vi "DllFxpAtan2Temp.vi"(6 "ready for output":bool, 9 "input valid":bool, 10 "x":fxp<+/-,64,32>, 11 "y":fxp<+/-,64,32>) -> (1 "output valid":bool, 3 "atan2(y, x)":fxp<+,1,1>, 4 "ready for input":bool)   [LabVIEW 2017]
uses:
  <vilib>/rvi/FXPMathLib/FxpAtan2/subVIs/nifxpmath_Atan2_SimConfig.ctl
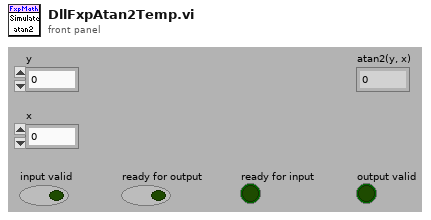
[diagram p1: front panel]
types:
  T1 = typedef "nifxpmath_Atan2_SimConfig.ctl" = cluster{"kXSigned":bool, "kXWl":u32, "kXIwl":i32, "kYSigned":bool, "kYWl":u32, "kYIwl":i32, "kAtan2Signed":bool, "kAtan2Wl":u32, "kAtan2Iwl":i32, "internal xy wl":u16, "internal xy iwl":i16, "kCoarseRotation":bool, "kPrecision":u16, "kIteration":u16, "kQuaMode":u16, "kInsideSCTL":bool, "CycleLimit":u16, "StrictLimit":bool, "InputRegister":bool, "OutputRegister":bool}
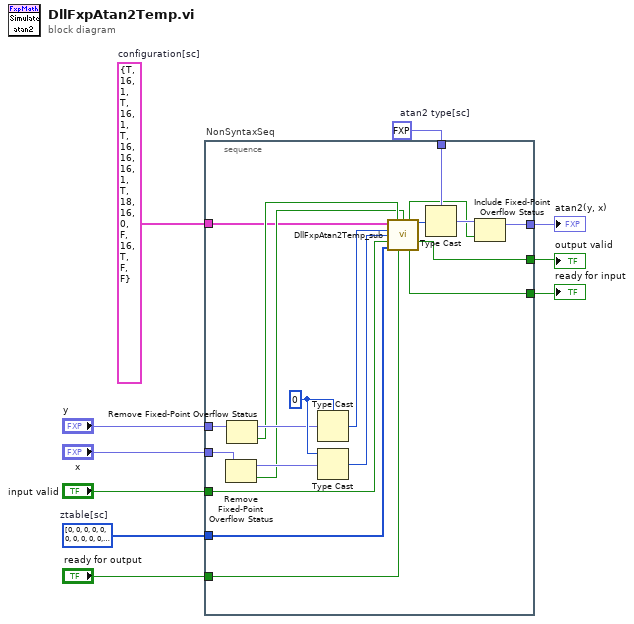
[diagram p0: block diagram]
diagram:
  w1 = T1 {"kXSigned"=TRUE, "kXWl"=16, "kXIwl"=1, "kYSigned"=TRUE, "kYWl"=16, "kYIwl"=1, "kAtan2Signed"=TRUE, "kAtan2Wl"=16, "kAtan2Iwl"=16, "internal xy wl"=16, "internal xy iwl"=1, "kCoarseRotation"=TRUE, "kPrecision"=18, "kIteration"=16, "kQuaMode"=0, "kInsideSCTL"=FALSE, "CycleLimit"=16, "StrictLimit"=TRUE, "InputRegister"=FALSE, "OutputRegister"=FALSE}  # configuration[sc]
  w5 = fxp<+,1,1> 0.0  # atan2 type[sc]
  w6 = u64[] [0, 0, 0, 0, 0, 0, 0, 0, 0, 0, 0, 0, 0, 0, 0, 0, 0, 0]  # ztable[sc]
  n1 = stacked-sequence "NonSyntaxSeq" {
    tunnel: "y" -> [w28]
    tunnel: "input valid" -> [w16]
    tunnel: [w19] -> w8
    tunnel: "x" -> [w27]
    tunnel: w6 -> [w15]
    tunnel: w5 -> [w29]
    tunnel: "ready for output" -> [w14]
    tunnel: [w13] -> w3
    tunnel: [w12] -> w2
    tunnel: w1 -> [w11]
    frame #0 {
      w30 = u64 0
      n2 = Remove Fixed-Point Overflow Status(3:w27) -> (0:w23:bool, 1:w25:fxp<+/-,64,32>)
      n3 = Remove Fixed-Point Overflow Status(3:w28) -> (0:w24:bool, 1:w26:fxp<+/-,64,32>)
      n4 = Type Cast(type=w30, x=w26) -> (*(type *) &x=w18:u64)
      n5 = Type Cast(type=w30, x=w25) -> (*(type *) &x=w17:u64)
      n6 = call <vilib>:"DllFxpAtan2Temp_sub.vi"("configuration[sc]"=w11, "y ovfl status"=w24, "x ovfl status"=w23, "y"=w18, "x"=w17, "input valid"=w16, "ztable"=w15, "ready for output"=w14) -> ("atan2 ovfl status"=w20:bool, "atan2(y, x)"=w22:u64, "output valid"=w13:bool, "ready for input"=w12:bool)  [unwired: 4 out]
      n7 = Type Cast(type=w29, x=w22) -> (*(type *) &x=w21:fxp<+,1,1>)
      n8 = Include Fixed-Point Overflow Status(2:w20, 3:w21) -> (1:w19:fxp<+,1,1>)
    }
  }
  "atan2(y, x)" <- w8
  "output valid" <- w3
  "ready for input" <- w2
